vi "_Main_04.vi"() -> ()   [LabVIEW 2017]
uses:
  <vilib>/Instr/_visa.llb/VISA Configure Serial Port (Instr).vi
panel:
  out "Boolean 2":bool
  in  "Speed, K/min":dbl=5.0 min=0.1 max=10.0
  in  "Target, K":dbl=295.0 min=195.0 max=395.0
  in  "Ramp":bool
  out "tempC":dbl format="%#.2g"
  out "Power LOG":cluster{dbl[], dbl[]}(graph)
  in  "Boolean":bool
  out "y":dbl
  in  "Set temp":dbl=195.0 min=195.0 max=395.0
  in  "Setpoint":bool
  out "TrigTimer, s":dbl
  out "tempK":dbl format="%#.2g"
  out "serv1":i32
  out "serv2":i32
  out "serv3":i32
  out "serv4":i32
  out "Vout, V":dbl format="%#.2g"
  out "Vin, V":dbl format="%#.5g"
  out "Temp, K":dbl
  out "Temp_sp, K":dbl
  out "Temp_gsp, K":dbl
  out "Temp LOG":cluster{dbl[], dbl[]}(graph)
  out "Bytes at Port":u32
  out "RecTry":i32
  in  "Stop Button":bool
  in  "COM port":refnum<visa-resource-name>
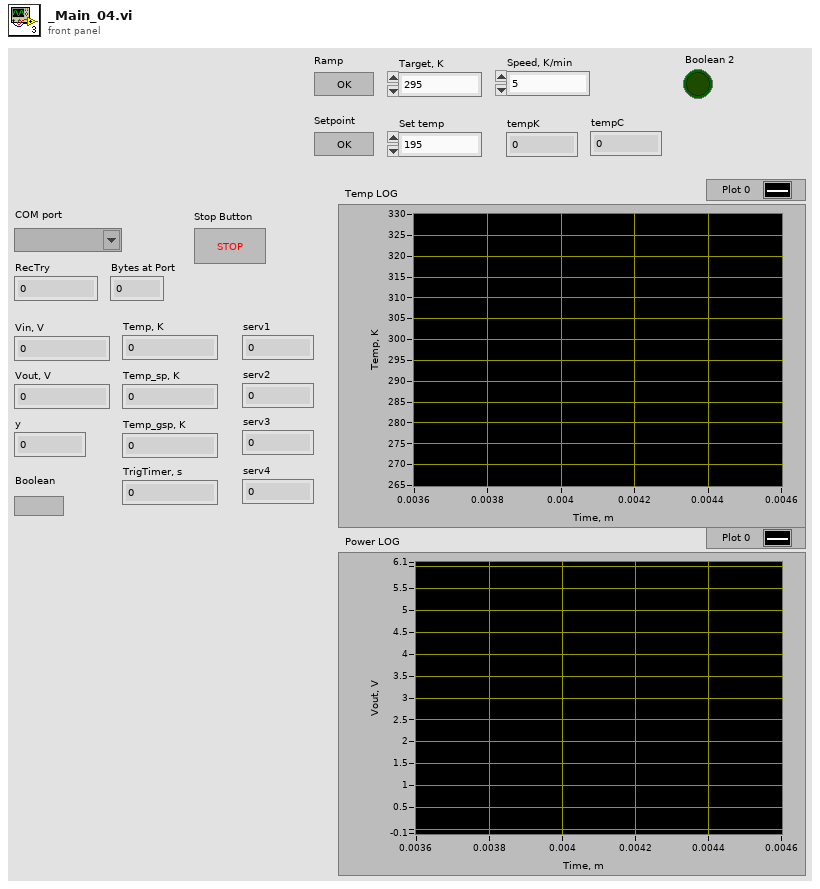
[diagram p1: front panel]
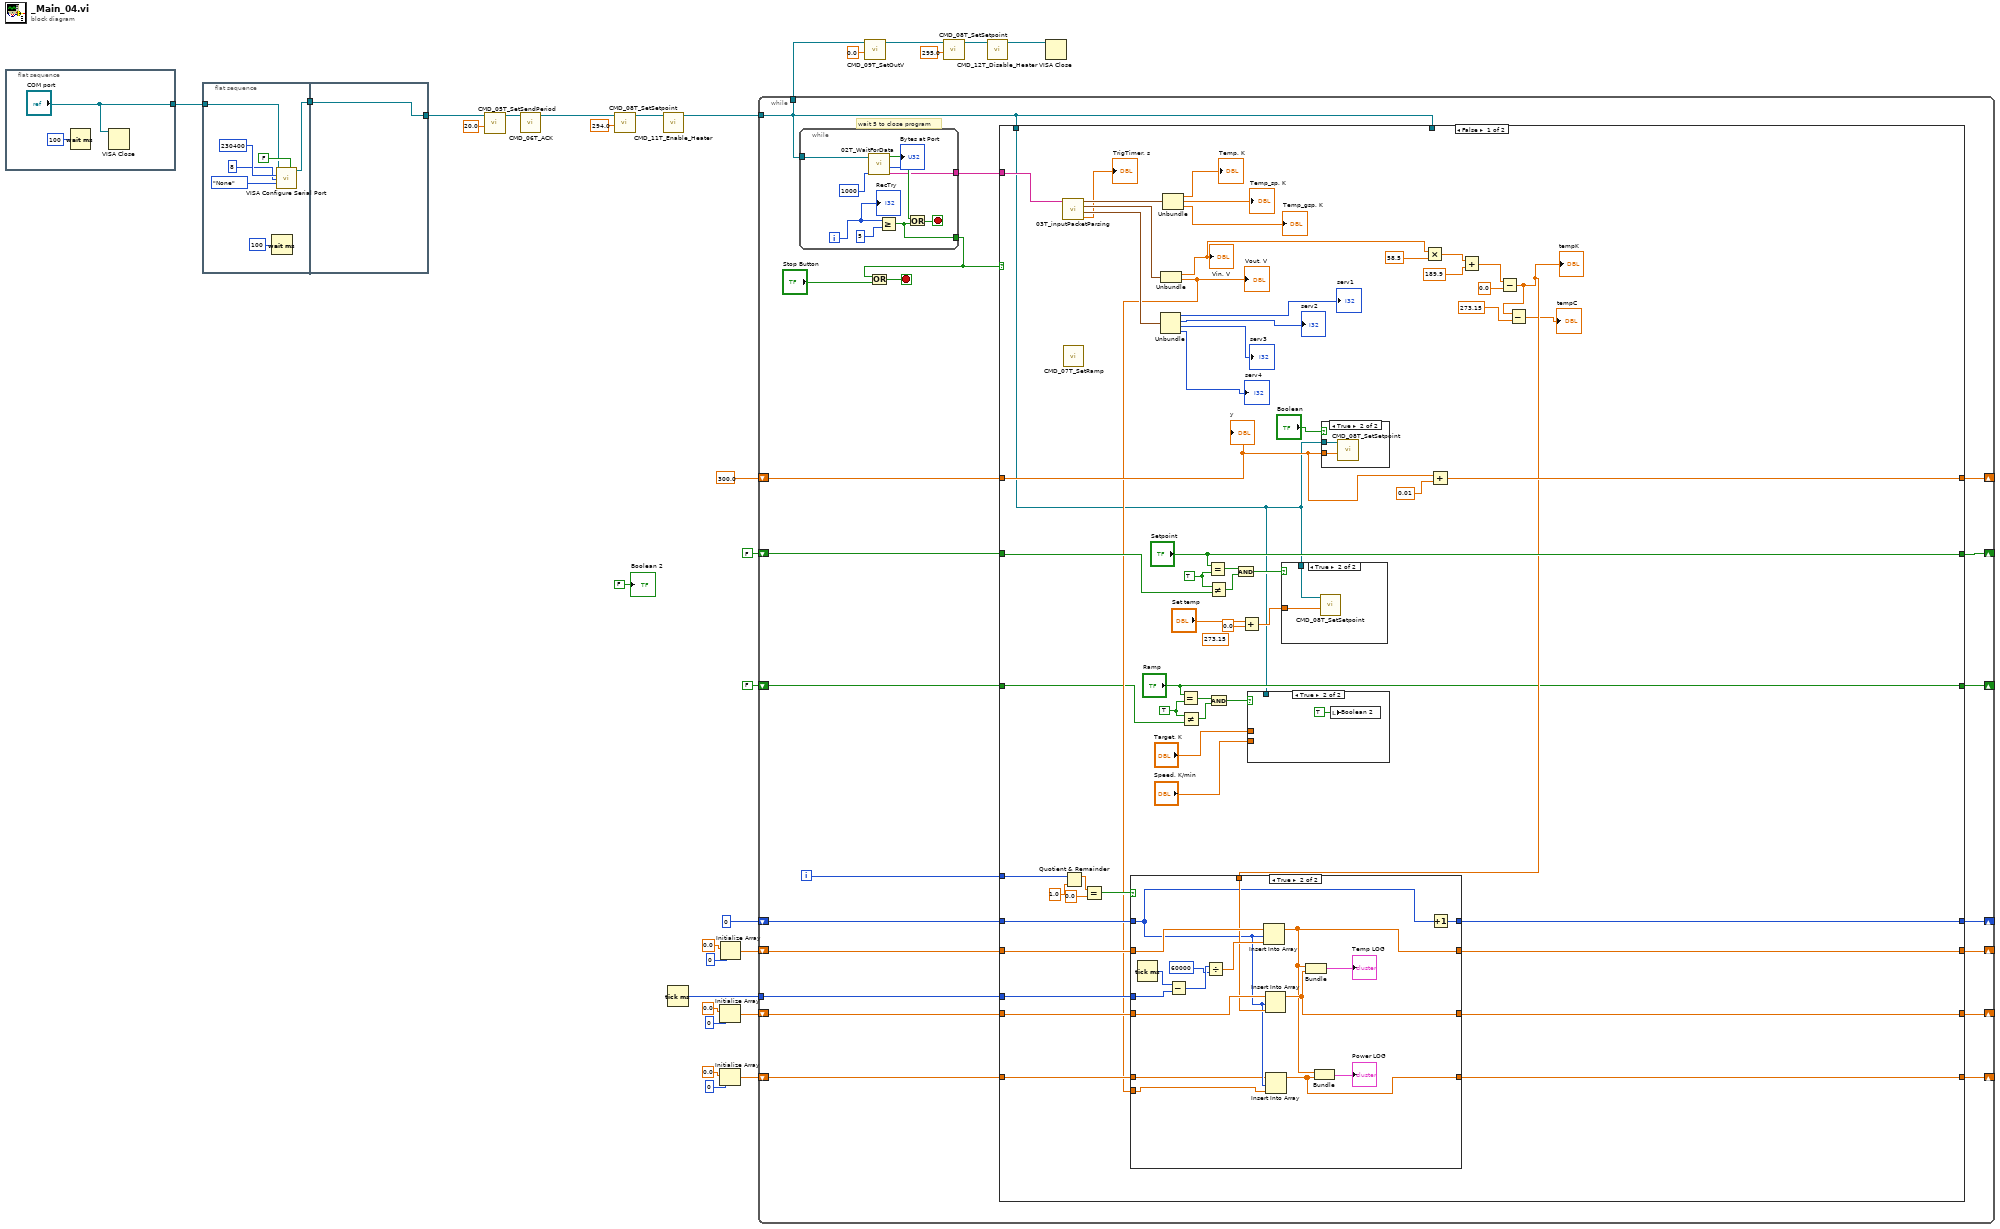
[diagram p0: block diagram]
diagram:
  n1 = flat-sequence {
    tunnel: ["COM port"] -> w30
    frame #0 {
      n2 = Wait (ms)(milliseconds to wait=u32 100) -> ()  [unwired: 1 out]
      n3 = VISA Close(VISA resource name="COM port") -> ()  [unwired: 1 in, 1 out]
    }
  }
  n4 = flat-sequence {
    tunnel: w30 -> [w35]
    tunnel: [w34] -> w27
    tunnel: [w40] -> w18
    tunnel: w27 -> [w40]
    frame #0 {
      n5 = Wait (ms)(milliseconds to wait=u32 100) -> ()  [unwired: 1 out]
      n6 = call-poly "VISA Configure Serial Port"("VISA resource name"=w35, "Enable Termination\nChar (T)"=FALSE ("Enable Termination\nChar (T)"), "baud rate (9600)"=u32 230400, "data bits (8)"=u16 8, "parity (0:none)"=enum16{"None", "Odd", "Even", "Mark", "Space"}."None") -> ("VISA resource name out"=w34:refnum<visa-resource-name>)  [unwired: 9 in, 1 out]
    }
    frame #1 {
    }
  }
  n7 = call "CMD_05T_SetSendPeriod.vi"("Period, ms"=20.0, "VISA resource name"=w18) -> ("VISA resource name out"=w28:refnum<visa-resource-name>)  [unwired: 9 in]
  n8 = call "CMD_06T_ACK.vi"("VISA resource name"=w28) -> ("VISA resource name out"=w7:refnum<visa-resource-name>)  [unwired: 10 in]
  n9 = call "CMD_08T_SetSetpoint.vi"("Setpoint, K"=294.0, "VISA resource name"=w7) -> ("VISA resource name out"=w4:refnum<visa-resource-name>)  [unwired: 9 in]
  n10 = call "CMD_11T_Enable_Heater.vi"("VISA resource name"=w4) -> ("VISA resource name out"=w3:refnum<visa-resource-name>)  [unwired: 10 in]
  n11 = Tick Count (ms)() -> (millisecond timer value=w22:u32)
  n12 = Initialize Array(0.0 ("element"), 0 ("dimension size")) -> (w19:dbl[])
  n13 = Initialize Array(0.0 ("element"), 0 ("dimension size")) -> (w8:dbl[])
  n14 = Initialize Array(0.0 ("element"), 0 ("dimension size")) -> (w23:dbl[])
  n15 = while {
    tunnel: w3 -> [w47]
    tunnel: [w47] -> w17
    shift-right: [w56] -> _
    shift-left: 0 -> [w57]
    tunnel: w22 -> [w54]
    shift-right: [w52] -> _
    shift-left: w23 -> [w55]
    shift-right: [w51] -> _
    shift-left: w19 -> [w53]
    shift-right: [w49] -> _
    shift-left: FALSE ("OK Button") -> [w48]
    shift-right: [w45] -> _
    shift-left: 300.0 ("y") -> [w46]
    shift-right: [w43] -> _
    shift-left: w8 -> [w44]
    shift-right: [w42] -> _
    shift-left: FALSE ("Ramp") -> [w41]
    i -> [w58]
    stop <- w61 stop-if-true
    # "wait 5 to close program"
    n16 = while {
      tunnel: w47 -> [w153]
      tunnel: [w156] -> w60
      tunnel: [w157] -> w59
      i -> [w155]
      stop <- w159 stop-if-true
      n17 = call "02T_WaitForData.vi"("WaitTimeoutMS"=u32 1000, "VISA"=w153) -> ("Buffer"=w157:string, "Bytes at Port"=→"Bytes at Port":u32, "Data Recived"=w158:bool)  [unwired: 7 in]
      n18 = Greater Or Equal?(x=w155, y=5) -> (x >= y?=w156:bool)
      n19 = Or(x=w158, y=w156) -> (x .or. y?=w159:bool)
      "RecTry" <- w155
    }
    n20 = Or(x=w60, y="Stop Button") -> (x .or. y?=w61:bool)
    n21 = case shown="False" w60 {
      tunnel: w59 -> [w110 _]
      tunnel: w58 -> [w116 _]
      tunnel: w47 -> [_ _]
      tunnel: w57 -> [w114 w152]
      tunnel: [w113 w152] -> w56
      tunnel: w55 -> [w98 w151]
      tunnel: w54 -> [w112 _]
      tunnel: w53 -> [w96 w150]
      tunnel: [w111 w151] -> w52
      tunnel: [w89 w150] -> w51
      tunnel: ["Setpoint" w149] -> w49
      tunnel: w48 -> [w93 w149]
      tunnel: w47 -> [w64 _]
      tunnel: w46 -> [w83 w148]
      tunnel: [w84 w148] -> w45
      tunnel: w44 -> [w80 w147]
      tunnel: [w79 w147] -> w43
      tunnel: ["Ramp" w146] -> w42
      tunnel: w41 -> [w66 w146]
      frame False {
        w67 = TRUE ("y")
        (unwired) 273.15 ("y")
        w92 = TRUE ("x")
        n22 = call "03T_inputPacketParsing.vi"("string"=w110) -> ("TrigTimer, s"=→"TrigTimer, s":dbl, "Service"=w104:cluster{i32, i32, i32, i32}, "Voltage"=w105:cluster{dbl, dbl}, "Temp"=w109:cluster{dbl, dbl, dbl})  [unwired: 7 in]
        n23 = call "CMD_07T_SetRamp.vi"() -> ()  [unwired: 11 in, 1 out]
        n24 = Quotient & Remainder(x=w116, y=1.0) -> (x-y*floor(x/y)=w119:dbl)  [unwired: 1 out]
        n25 = Equal?(x=w119, y=0.0) -> (x = y?=w115:bool)
        n26 = Unbundle(w104) -> (→"serv1":i32, →"serv2":i32, →"serv3":i32, →"serv4":i32)
        n27 = Unbundle(w105) -> (w103:dbl, w78:dbl)
        "Vin, V" <- w103
        "Vout, V" <- w78
        n28 = Unbundle(w109) -> (→"Temp, K":dbl, →"Temp_sp, K":dbl, →"Temp_gsp, K":dbl)
        n29 = Equal?(x="Ramp", y=w67) -> (x = y?=w70:bool)
        n30 = Not Equal?(x=w67, y=w66) -> (x != y?=w69:bool)
        n31 = Equal?(x="Setpoint", y=w92) -> (x = y?=w95:bool)
        n32 = Not Equal?(x=w92, y=w93) -> (x != y?=w91:bool)
        n33 = And(x=w70, y=w69) -> (x .and. y?=w65:bool)
        n34 = And(x=w95, y=w91) -> (x .and. y?=w90:bool)
        n35 = Add(x="Set temp", y=0.0) -> (x+y=w88:dbl)
        n36 = case shown="True" w65 {
          tunnel: w64 -> [_ _]
          tunnel: "Target, K" -> [_ _]
          tunnel: "Speed, K/min" -> [_ _]
          frame False {
          }
          frame True {
            n37 = local write "Boolean 2"(TRUE ("Boolean 2")) -> ()
          }
        }
        n38 = case shown="True" w90 {
          tunnel: w88 -> [_ w124]
          tunnel: w64 -> [_ w123]
          frame False {
          }
          frame True {
            n39 = call "CMD_08T_SetSetpoint.vi"("Setpoint, K"=w124, "VISA resource name"=w123) -> ()  [unwired: 9 in, 1 out]
          }
        }
        n40 = case shown="True" "Boolean" {
          tunnel: w64 -> [_ w122]
          tunnel: w83 -> [_ w121]
          frame False {
          }
          frame True {
            n41 = call "CMD_08T_SetSetpoint.vi"("Setpoint, K"=w121, "VISA resource name"=w122) -> ()  [unwired: 9 in, 1 out]
          }
        }
        n42 = Multiply(x=w103, y=58.5) -> (x*y=w101:dbl)
        n43 = Add(x=w83, y=0.01) -> (x+y=w84:dbl)
        n44 = Add(x=w101, y=189.9) -> (x+y=w99:dbl)
        n45 = Subtract(x=w99, y=0.0) -> (x-y=w77:dbl)
        "tempK" <- w77
        n46 = case shown="True" w115 {
          tunnel: w114 -> [w128 w134]
          tunnel: [w128 w141] -> w113
          tunnel: w98 -> [w126 w139]
          tunnel: w112 -> [_ w144]
          tunnel: w96 -> [w127 w138]
          tunnel: [w127 w136] -> w89
          tunnel: [w126 w132] -> w111
          tunnel: w77 -> [_ w135]
          tunnel: w80 -> [w125 w133]
          tunnel: [w125 w130] -> w79
          tunnel: w78 -> [_ w129]
          frame False {
          }
          frame True {
            n47 = Tick Count (ms)() -> (millisecond timer value=w145:u32)
            n48 = Subtract(x=w145, y=w144) -> (x-y=w143:u32)
            n49 = Divide(x=w143, y=u32 60000) -> (x/y=w140:dbl)
            n50 = Insert Into Array(array=w139, index=w134, new element=w140) -> (w132:dbl[])
            n51 = Insert Into Array(array=w138, index=w134, new element=w135) -> (w136:dbl[])
            n52 = Insert Into Array(array=w133, index=w134, new element=w129) -> (w130:dbl[])
            n53 = Bundle(w132, w136) -> (→"Temp LOG":cluster{dbl[], dbl[]})  [unwired: 1 in]
            n54 = Bundle(w132, w130) -> (→"Power LOG":cluster{dbl[], dbl[]})  [unwired: 1 in]
            n55 = Increment(x=w134) -> (x+1=w141:i32)
          }
        }
        n56 = Subtract(x=w77, y=273.15) -> (x-y=→"tempC":dbl)
        "y" <- w83
      }
      frame True {
      }
    }
  }
  n57 = call "CMD_09T_SetOutV.vi"("Voltage, d"=0.0, "VISA resource name"=w17) -> ("VISA resource name out"=w12:refnum<visa-resource-name>)  [unwired: 9 in]
  n58 = call "CMD_08T_SetSetpoint.vi"("Setpoint, K"=295.0, "VISA resource name"=w12) -> ("VISA resource name out"=w6:refnum<visa-resource-name>)  [unwired: 9 in]
  n59 = call "CMD_12T_Disable_Heater.vi"("VISA resource name"=w6) -> ("VISA resource name out"=w5:refnum<visa-resource-name>)  [unwired: 10 in]
  n60 = VISA Close(VISA resource name=w5) -> ()  [unwired: 1 in, 1 out]
  "Boolean 2" <- FALSE ("Boolean 2")
